vi "Merge Tests.vi"() -> ()   [LabVIEW 2020]
uses:
  Column Configuration.lvclass
  Database Libraries/ADODB/ADODB Class/ADODB.lvclass
  C:/Users/User/Desktop/Raman Program/LV-Database-OOP/source/Database OOP/Database Libraries/Database Interfaces/Database Interface Class/Database Interface.lvclass
  Database Libraries/Database Interfaces/Database data type.ctl
  Database Libraries/Database Interfaces.lvlib
panel:
  out "Merge default over non-default config passed":bool
  out "Merge over default config passed":bool
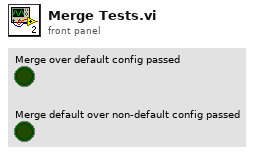
[diagram p1: front panel]
types:
  T1 = typedef "Database Interfaces.lvlib/Database data type.ctl" = enum16{"Undefined", "String", "Long (I32)", "Single (SGL)", "Double (DBL)", "Date/Time", "Binary"}
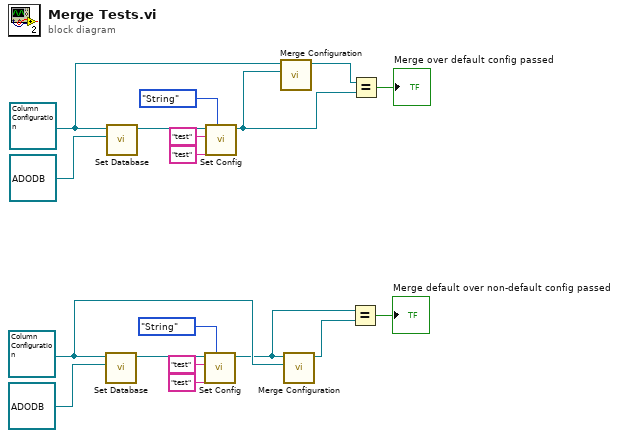
[diagram p0: block diagram]
diagram:
  w3 = refnum<class "Column Configuration.lvclass"> refnum ("Column Configuration in")
  w4 = refnum<class "Column Configuration.lvclass"> refnum ("Column Configuration in")
  n1 = call-dynamic "Set Database.vi"("Database"=refnum<class "ADODB.lvclass"> refnum ("ADODB.lvlib:ADODB.lvclass"), "Basic Column Configuration in"=w3) -> ("Basic Column Configuration out"=w6:refnum<class "Column Configuration.lvclass">)  [unwired: 8 in, 1 out]
  n2 = call-dynamic "Set Database.vi"("Database"=refnum<class "ADODB.lvclass"> refnum ("ADODB.lvlib:ADODB.lvclass"), "Basic Column Configuration in"=w4) -> ("Basic Column Configuration out"=w17:refnum<class "Column Configuration.lvclass">)  [unwired: 8 in, 1 out]
  n3 = call "Set Config.vi"("Column Type"=Database_data_type."String", "Column Name"="test", "Table Name"="test", "Basic Column Configuration in"=w6) -> ("Basic Column Configuration out"=w1:refnum<class "Column Configuration.lvclass">)  [unwired: 6 in, 1 out]
  n4 = call "Set Config.vi"("Column Type"=Database_data_type."String", "Column Name"="test", "Table Name"="test", "Basic Column Configuration in"=w17) -> ("Basic Column Configuration out"=w12:refnum<class "Column Configuration.lvclass">)  [unwired: 6 in, 1 out]
  n5 = call-dynamic "Merge Configuration.vi"("Configuration to Merge"=w12, "Column Configuration in"=w4) -> ("Column Configuration out"=w13:refnum<class "Column Configuration.lvclass">)  [unwired: 8 in, 1 out]
  n6 = call-dynamic "Merge Configuration.vi"("Configuration to Merge"=w3, "Column Configuration in"=w1) -> ("Column Configuration out"=w2:refnum<class "Column Configuration.lvclass">)  [unwired: 8 in, 1 out]
  n7 = Equal?(x=w1, y=w2) -> (x = y?=→"Merge default over non-default config passed":bool)
  n8 = Equal?(x=w13, y=w12) -> (x = y?=→"Merge over default config passed":bool)
